vi "Get Owning Path Default Value.vi"(0 "SG Path Group in":refnum<class "SG 8GHz Path Group.lvclass">, 11 "error in":errorcluster) -> (4 "SG Path Group out":refnum<class "SG 8GHz Path Group.lvclass">, 6 "Path":refnum<class "Path.lvclass">, 15 "error out":errorcluster)   [LabVIEW 2023, in "RFFixtureCharact.RMM.lvlib" / "SG 8GHz Path Group.lvclass"]
uses:
  Common/Base Classes/Path/Path.lvclass
  SG 8GHz Path Group.lvclass
  SG 8GHz Path Group.lvclass/SG 8GHz Path Group.ctl
  Paths/SG 8GHz Path/SG 8GHz Path.lvclass
  C:/srd-semi-rfcal-software/AuxTools/STSRFFixtureCharactUtility/Source/Code Modules/Fixture/Public/Base Classes/Scalar/SG Path/SG Path.lvclass
  C:/srd-semi-rfcal-software/AuxTools/STSRFFixtureCharactUtility/Source/Code Modules/Fixture/Public/Base Classes/Scalar/SG Abstract Path/SG Abstract Path.lvclass
  C:/srd-semi-rfcal-software/AuxTools/STSRFFixtureCharactUtility/Source/Code Modules/Fixture/Public/Base Classes/Scalar/Scalar Path/Scalar Path.lvclass
  C:/srd-semi-rfcal-software/AuxTools/STSRFFixtureCharactUtility/Source/Code Modules/Common/Base Classes/Path/Path.lvclass
  C:/srd-semi-rfcal-software/AuxTools/STSRFFixtureCharactUtility/Source/Code Modules/Fixture/RMM/Scalar/Paths/SG 8GHz Path/SG 8GHz Path.lvclass
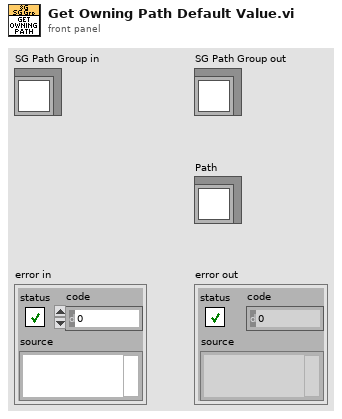
[diagram p1: front panel]
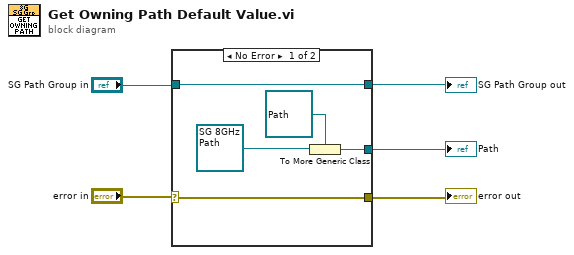
[diagram p0: block diagram]
diagram:
  n1 = case shown="No Error" "error in" {
    selector: "error in" -> [w10 w11]
    tunnel: [w7 _] -> w3
    tunnel: [w10 w11] -> w2
    tunnel: [w9 w12] -> w5
    tunnel: "SG Path Group in" -> [w9 w12]
    frame No Error {
      n2 = To More Generic Class(target class=refnum<class "Path.lvclass"> refnum ("Path"), reference=refnum<class "SG 8GHz Path.lvclass"> refnum ("SG 8GHz Path.lvclass")) -> (generic class reference=w7:refnum<class "Path.lvclass">)
    }
    frame Error {
    }
  }
  "error out" <- w2
  "SG Path Group out" <- w5
  "Path" <- w3
